vi "Remove All Keys.vi"(8 "error in":errorcluster, 11 "E2E configuration in":refnum<class "E2E Tag Exchange configuration.lvclass">) -> (0 "error out":errorcluster, 3 "E2E configuration out":refnum<class "E2E Tag Exchange configuration.lvclass">)   [LabVIEW 2015, in "E2E Tag Exchange configuration.lvclass"]
uses:
  E2E Tag Exchange configuration.lvclass
  E2E Tag Exchange configuration.lvclass/E2E Tag Exchange configuration.ctl
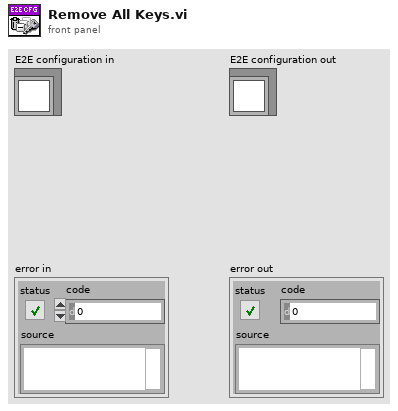
[diagram p1: front panel]
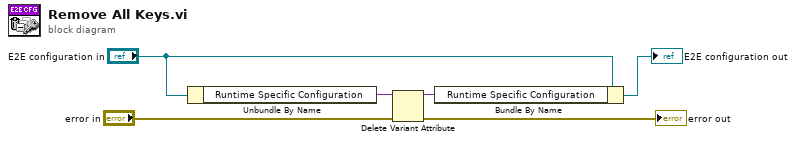
[diagram p0: block diagram]
diagram:
  n1 = Unbundle By Name("E2E configuration in") -> ("Runtime Specific Configuration"=w1:variant)
  n2 = Delete Variant Attribute(4:"error in", 7:w1) -> (0:→"error out":errorcluster, 3:w5:variant)  [unwired: 1 in, 1 out]
  n3 = Bundle By Name(cluster="E2E configuration in", "Runtime Specific Configuration"=w5) -> (→"E2E configuration out":refnum<class "E2E Tag Exchange configuration.lvclass">)
